vi "Main.vi"() -> ()   [LabVIEW 2019]
panel:
  in  "?":T1
  out "?":string
  # "Casio-VI/001"
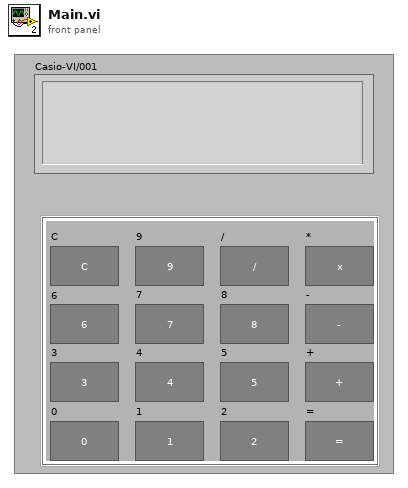
[diagram p1: front panel]
types:
  T1 = cluster{cluster{"2":bool, "1":bool, "0":bool, "3":bool, "5":bool, "4":bool, "7":bool, "6":bool, "8":bool, "+":bool, "9":bool, "*":bool, "-":bool, "/":bool, "=":bool, "C":bool}}
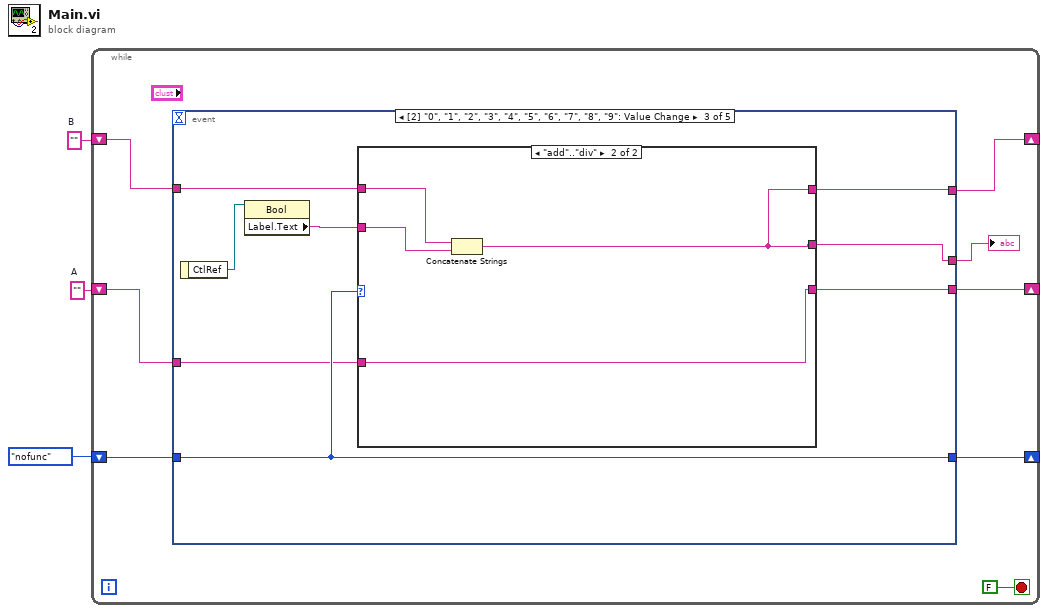
[diagram p0: block diagram]
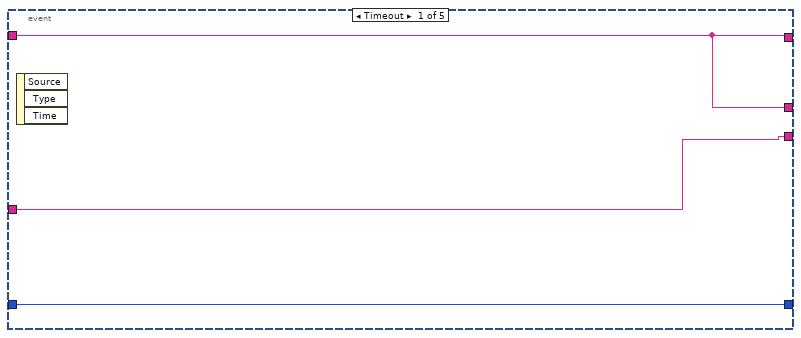
[diagram p2: hidden frame]
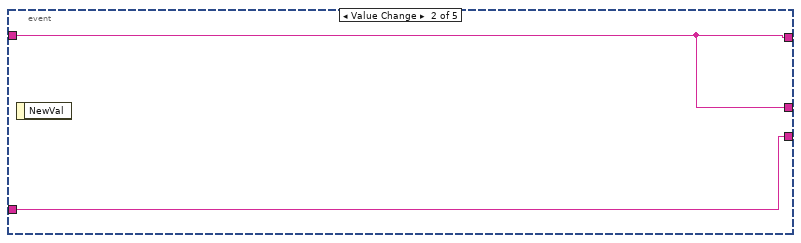
[diagram p3: hidden frame]
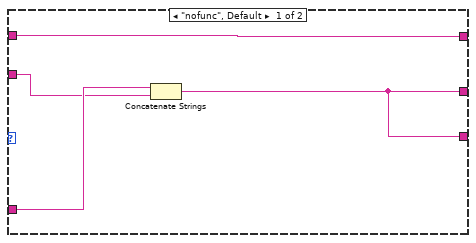
[diagram p4: hidden frame]
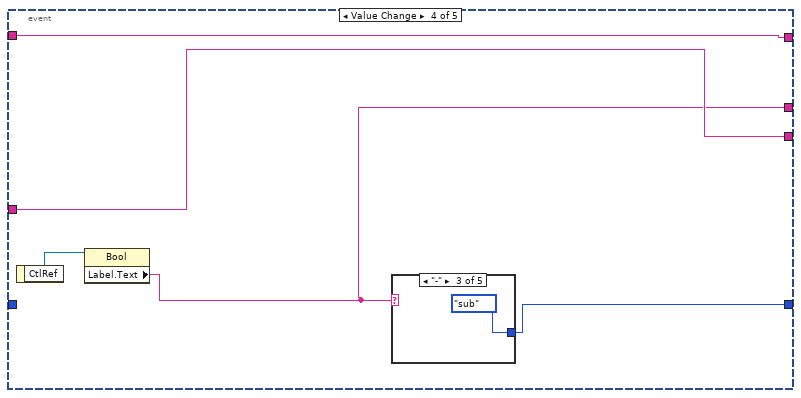
[diagram p5: hidden frame]
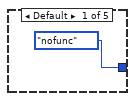
[diagram p6: hidden frame]
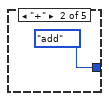
[diagram p7: hidden frame]
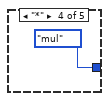
[diagram p8: hidden frame]
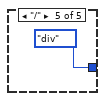
[diagram p9: hidden frame]
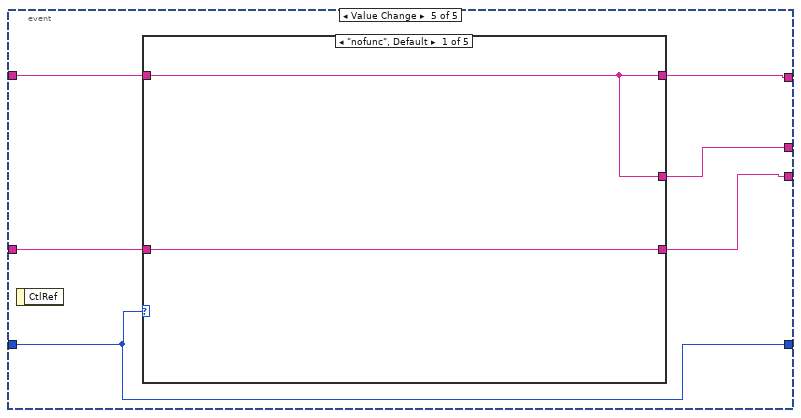
[diagram p10: hidden frame]
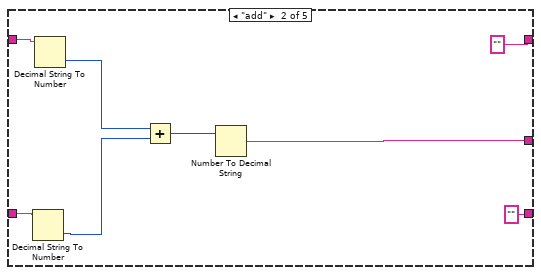
[diagram p11: hidden frame]
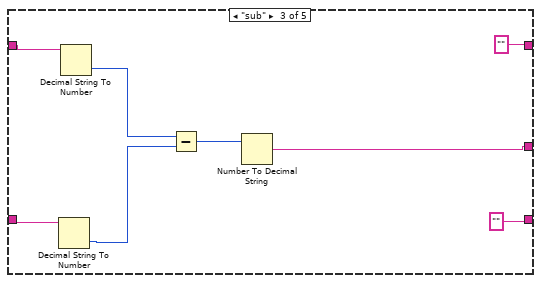
[diagram p12: hidden frame]
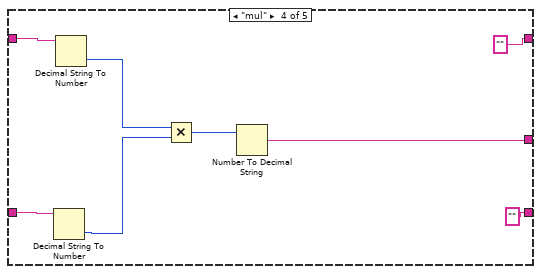
[diagram p13: hidden frame]
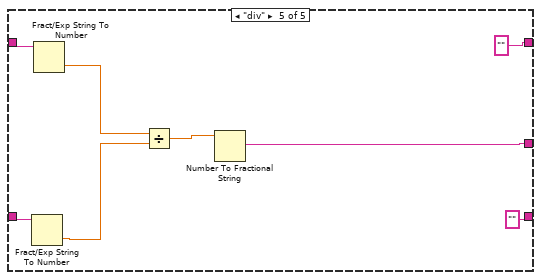
[diagram p14: hidden frame]
diagram:
  w3 = ""  # A
  w1 = ""  # B
  n1 = while {
    shift-right: [w6] -> _
    shift-left: w1 -> [w11]
    shift-right: [w7] -> _
    shift-left: w3 -> [w10]
    shift-right: [w8] -> _
    shift-left: enum16{"nofunc", "add", "sub", "mul", "div"}."nofunc" -> [w9]
    stop <- FALSE stop-if-true
    n2 = event shown="[2] \"0\", \"1\", \"2\", \"3\", \"4\", \"5\", \"6\", \"7\", \"8\", \"9\": Value Change" {
      selector: _ -> [_ _ _ _ _]
      dyn-events: _ -> [_ _ _ _ _]
      timeout: _ -> [_ _ _ _ _]
      tunnel: w11 -> [w12 w16 w18 w36 w47]
      tunnel: w10 -> [w14 w15 w21 w35 w46]
      tunnel: w9 -> [w13 _ w23 _ w48]
      tunnel: [w13 _ w23 w34 w48] -> w8
      tunnel: [w14 w15 w19 w35 w45] -> w7
      tunnel: [w12 w16 w17 w36 w44] -> w6
      tunnel: [w12 w16 w20 w33 w43] -> w5
      event Timeout {
        n3 = event-data() -> ()  [unwired: 1 in, 3 out]
      }
      event Value Change {
        n4 = event-data() -> ()  [unwired: 1 in, 1 out]
      }
      event Value Change {
        n5 = event-data() -> ("CtlRef"=w24:refnum<vi>)  [unwired: 1 in]
        n6 = property class="Bool"(reference=w24) -> ("Label.Text"=w22:string)  [unwired: 1 in, 2 out]
        n7 = case shown="\"add\"..\"div\"" w23 {
          tunnel: w22 -> [w27 w32]
          tunnel: w21 -> [w28 w29]
          tunnel: [w26 w30] -> w20
          tunnel: [w26 w29] -> w19
          tunnel: w18 -> [w25 w31]
          tunnel: [w25 w30] -> w17
          frame "nofunc", Default {
            n8 = Concatenate Strings(w28, w27) -> (w26:string)
          }
          frame "add".."div" {
            n9 = Concatenate Strings(w31, w32) -> (w30:string)
          }
        }
      }
      event Value Change {
        n10 = event-data() -> ("CtlRef"=w37:refnum<vi>)  [unwired: 1 in]
        n11 = property class="Bool"(reference=w37) -> ("Label.Text"=w33:string)  [unwired: 1 in, 2 out]
        n12 = case shown="\"-\"" w33 {
          tunnel: [enum16{"nofunc", "add", "sub", "mul", "div"}."nofunc" enum16{"nofunc", "add", "sub", "mul", "div"}."add" enum16{"nofunc", "add", "sub", "mul", "div"}."sub" enum16{"nofunc", "add", "sub", "mul", "div"}."mul" enum16{"nofunc", "add", "sub", "mul", "div"}."div"] -> w34
          frame Default {
          }
          frame "+" {
          }
          frame "-" {
          }
          frame "*" {
          }
          frame "/" {
          }
        }
      }
      event Value Change {
        n13 = event-data() -> ()  [unwired: 1 in, 1 out]
        n14 = case shown="\"nofunc\", Default" w48 {
          tunnel: w47 -> [w49 w58 w63 w70 w78]
          tunnel: w46 -> [w50 w57 w62 w69 w77]
          tunnel: [w49 "" "" "" ""] -> w44
          tunnel: [w50 "" "" "" ""] -> w45
          tunnel: [w49 w53 w61 w71 w79] -> w43
          frame "nofunc", Default {
          }
          frame "add" {
            n15 = Decimal String To Number(string=w57) -> (number=w55:i32)  [unwired: 2 in, 1 out]
            n16 = Decimal String To Number(string=w58) -> (number=w56:i32)  [unwired: 2 in, 1 out]
            n17 = Add(x=w56, y=w55) -> (x+y=w54:i32)
            n18 = Number To Decimal String(number=w54) -> (decimal integer string=w53:string)  [unwired: 1 in]
          }
          frame "sub" {
            n19 = Decimal String To Number(string=w62) -> (number=w65:i32)  [unwired: 2 in, 1 out]
            n20 = Decimal String To Number(string=w63) -> (number=w66:i32)  [unwired: 2 in, 1 out]
            n21 = Subtract(x=w66, y=w65) -> (x-y=w64:i32)
            n22 = Number To Decimal String(number=w64) -> (decimal integer string=w61:string)  [unwired: 1 in]
          }
          frame "mul" {
            n23 = Decimal String To Number(string=w69) -> (number=w73:i32)  [unwired: 2 in, 1 out]
            n24 = Decimal String To Number(string=w70) -> (number=w74:i32)  [unwired: 2 in, 1 out]
            n25 = Multiply(x=w74, y=w73) -> (x*y=w72:i32)
            n26 = Number To Decimal String(number=w72) -> (decimal integer string=w71:string)  [unwired: 1 in]
          }
          frame "div" {
            n27 = Fract/Exp String To Number(string=w77) -> (number=w81:dbl)  [unwired: 3 in, 1 out]
            n28 = Fract/Exp String To Number(string=w78) -> (number=w82:dbl)  [unwired: 3 in, 1 out]
            n29 = Divide(x=w82, y=w81) -> (x/y=w80:dbl)
            n30 = Number To Fractional String(number=w80) -> (F-format string=w79:string)  [unwired: 3 in]
          }
        }
      }
    }
    "?" <- w5
  }
